vi "update.vi"(8 "error in (no error)":errorcluster, 10 "adapter executability":T1={"instrument"=TRUE, "trajectory"=TRUE, "scanHead"=TRUE, "DAQ"=TRUE, "imageAssembler"=TRUE, "dataCollection"=TRUE, "display"=TRUE, "analyser"=TRUE, "stimulator"=TRUE}, 11 "ScanModeMG090624Camera in":refnum<class "ImagingModeMG090624Camera.lvclass">) -> (0 "error out":errorcluster, 3 "ScanModeMG090624Camera out":refnum<class "ImagingModeMG090624Camera.lvclass">)   [LabVIEW 2010, in "ImagingModeMG090624Camera.lvclass"]
uses:
  ImagingModeMG090624Camera.lvclass
  ImagingModeDL090923Scaffold/ImagingModeDL090923Scaffold/adapter_executability_cluster.ctl
  ImagingModeDL091001Scaffold/ImagingModeDL091001Scaffold/ImagingModeDL091001Scaffold.lvclass
  DAQ/GenericDAQ/GenericDAQ/GenericDAQ.lvclass
  ImageAssembler/GenericImageAssembler/GenericImageAssembler/GenericImageAssembler.lvclass
  DataCollection/GenericDataCollection/GenericDataCollection/GenericDataCollection.lvclass
  ImagingModeDL090923Scaffold/ImagingModeDL090923Scaffold/ImagingModeDL090923Scaffold.lvclass
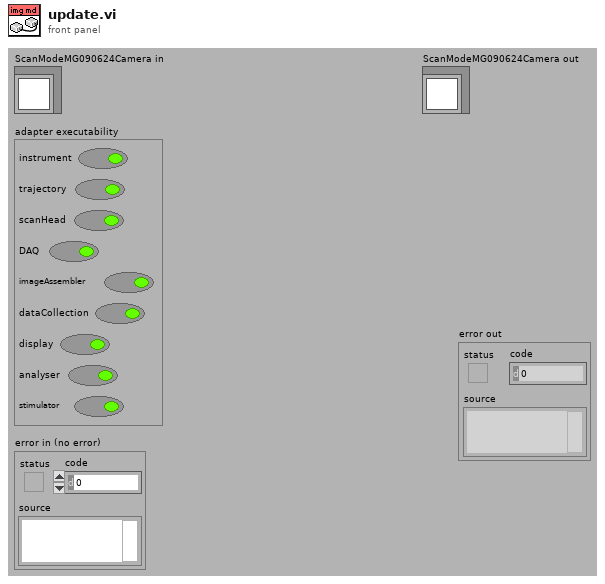
[diagram p1: front panel]
types:
  T1 = typedef "ImagingModeDL090923Scaffold.lvclass/adapter_executability_cluster.ctl" = cluster{"instrument":bool, "trajectory":bool, "scanHead":bool, "DAQ":bool, "imageAssembler":bool, "dataCollection":bool, "display":bool, "analyser":bool, "stimulator":bool}
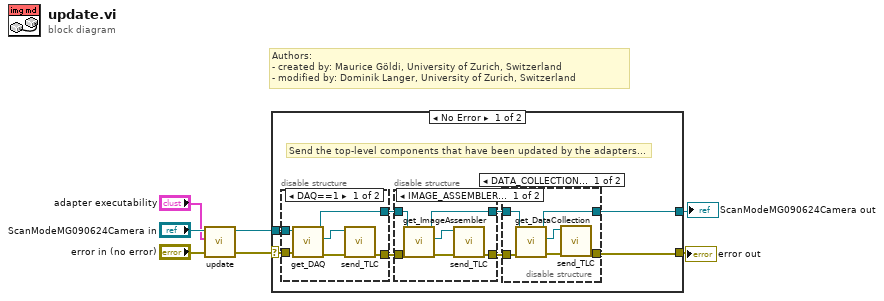
[diagram p0: block diagram]
diagram:
  # "Authors: \n- created by: Maurice Göldi, University of Zurich, Switzerland\n- modified by: Dominik Langer, University of Zurich, Switzerland"
  n1 = call-parent "update.vi"("error in (no error)"="error in (no error)", "adapter executability"="adapter executability", "ScanModeDL090923Scaffold in"="ScanModeMG090624Camera in") -> ("error out"=w4:errorcluster, "ScanModeDL090923Scaffold out"=w2:refnum<class "ImagingModeMG090624Camera.lvclass">)  [unwired: 7 in]
  n2 = case shown="No Error" w4 {
    selector: w4 -> [w11 w41]
    tunnel: [w15 w41] -> w7
    tunnel: [w12 w40] -> w6
    tunnel: w2 -> [w10 w40]
    frame No Error {
      # "Send the top-level components that have been updated by the adapters..."
      n3 = disable-structure shown="DAQ==1" {
        disable-tunnel: w11 -> [w36 w39]
        disable-tunnel: w10 -> [w35 w38]
        disable-tunnel: [w34 w39] -> w9
        disable-tunnel: [w32 w38] -> w8
        frame condition #0 (active) {
          n4 = call-dynamic "get_DAQ.vi"("error in (no error)"=w36, "ScanModeDL090923Scaffold in"=w35) -> ("error out"=w33:errorcluster, "DAQ"=w37:refnum<class "GenericDAQ.lvclass">, "ScanModeDL090923Scaffold out"=w32:refnum<class "ImagingModeMG090624Camera.lvclass">)  [unwired: 4 in, 3 out]
          n5 = call-dynamic "send_TLC.vi"("error in (no error)"=w33, "GenericToplevelComponent in"=w37) -> ("error out"=w34:errorcluster)  [unwired: 8 in, 1 out]
        }
        frame condition #1 {
        }
      }
      n6 = disable-structure shown="IMAGE_ASSEMBLER==1" {
        disable-tunnel: [w29 w31] -> w14
        disable-tunnel: [w27 w30] -> w13
        disable-tunnel: w9 -> [w26 w31]
        disable-tunnel: w8 -> [w25 w30]
        frame condition #0 (active) {
          n7 = call-dynamic "get_ImageAssembler.vi"("error in (no error)"=w26, "ScanModeDL090923Scaffold in"=w25) -> ("error out"=w28:errorcluster, "ImageAssembler"=w24:refnum<class "GenericImageAssembler.lvclass">, "ScanModeDL090923Scaffold out"=w27:refnum<class "ImagingModeMG090624Camera.lvclass">)  [unwired: 4 in, 3 out]
          n8 = call-dynamic "send_TLC.vi"("error in (no error)"=w28, "GenericToplevelComponent in"=w24) -> ("error out"=w29:errorcluster)  [unwired: 8 in, 1 out]
        }
        frame condition #1 {
        }
      }
      n9 = disable-structure shown="DATA_COLLECTION==1" {
        disable-tunnel: [w21 w23] -> w15
        disable-tunnel: w14 -> [w19 w23]
        disable-tunnel: w13 -> [w18 w22]
        disable-tunnel: [w16 w22] -> w12
        frame condition #0 (active) {
          n10 = call-dynamic "get_DataCollection.vi"("error in (no error)"=w19, "ScanModeDL090923Scaffold in"=w18) -> ("error out"=w20:errorcluster, "DataCollection"=w17:refnum<class "GenericDataCollection.lvclass">, "ScanModeDL090923Scaffold out"=w16:refnum<class "ImagingModeMG090624Camera.lvclass">)  [unwired: 4 in, 3 out]
          n11 = call-dynamic "send_TLC.vi"("error in (no error)"=w20, "GenericToplevelComponent in"=w17) -> ("error out"=w21:errorcluster)  [unwired: 8 in, 1 out]
        }
        frame condition #1 {
        }
      }
    }
    frame Error {
    }
  }
  "error out" <- w7
  "ScanModeMG090624Camera out" <- w6
